vi "Zad1_kolokwium.vi"() -> ()   [LabVIEW 2012]
panel:
  out "Wyrazy po彻czone w zdanie":string
  in  "wyraz 6":string
  in  "wyraz 5":string
  in  "wyraz 4":string
  in  "wyraz 3":string
  in  "wyraz 2":string
  in  "wyraz 1":string
  # "Program ³¹czy wpisane przez u¿ytkownika wyrazy w jedno zdanie"
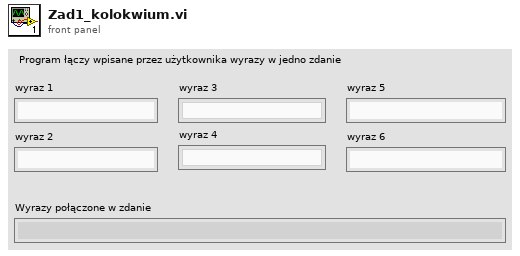
[diagram p1: front panel]
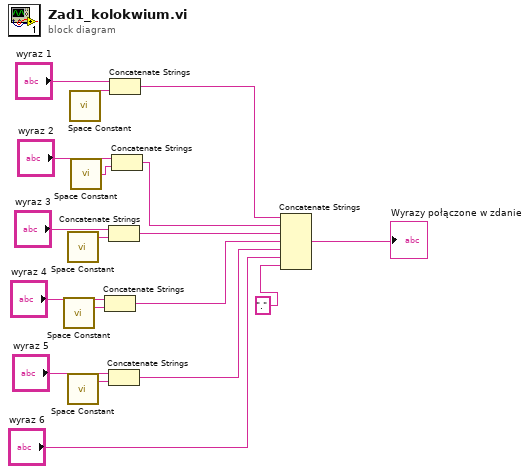
[diagram p0: block diagram]
diagram:
  n1 = call <vilib>:"Space Constant.vi"() -> ("String"=w11:string)
  n2 = call <vilib>:"Space Constant.vi"() -> ("String"=w13:string)
  n3 = call <vilib>:"Space Constant.vi"() -> ("String"=w9:string)
  n4 = call <vilib>:"Space Constant.vi"() -> ("String"=w17:string)
  n5 = call <vilib>:"Space Constant.vi"() -> ("String"=w15:string)
  n6 = Concatenate Strings("wyraz 4", w11) -> (w5:string)
  n7 = Concatenate Strings("wyraz 3", w13) -> (w6:string)
  n8 = Concatenate Strings("wyraz 5", w9) -> (w4:string)
  n9 = Concatenate Strings("wyraz 1", w17) -> (w8:string)
  n10 = Concatenate Strings("wyraz 2", w15) -> (w7:string)
  n11 = Concatenate Strings(w8, w7, w6, w5, w4, "wyraz 6", ".") -> (→"Wyrazy po彻czone w zdanie":string)
